vi "ABC Check Move Done.vi"(8 "UART":refnum<vi>, 9 "Response":string, 10 "DataIn":dbl[](array[numeric]), 11 "Data":refnum<vi>) -> (0 "Done":bool, 2 "DataOut":dbl[](array[numeric]), 4 "Position":dbl)   [LabVIEW 2020]
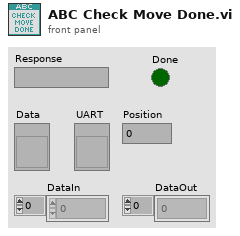
[diagram p1: front panel]
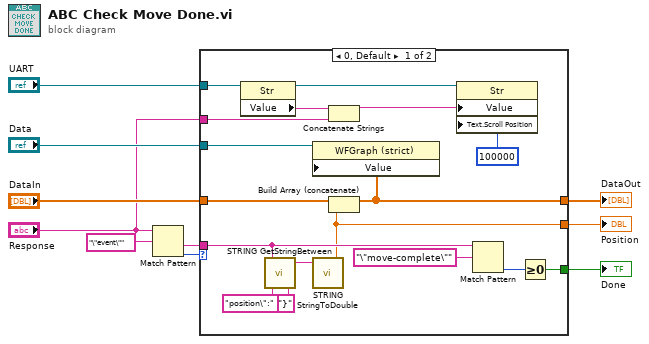
[diagram p0: block diagram]
diagram:
  n1 = Match Pattern(string="Response", regular expression="\"event\"") -> (after substring=w9:string, offset past match=w8:i32)  [unwired: 1 in, 2 out]
  n2 = case shown="0, Default" w8 {
    tunnel: w9 -> [w15 _]
    tunnel: "DataIn" -> [w24 w28]
    tunnel: [w22 w28] -> w6
    tunnel: "Data" -> [w23 _]
    tunnel: "UART" -> [w18 _]
    tunnel: [w14 _] -> w3
    tunnel: "Response" -> [w13 _]
    tunnel: [w11 _] -> w1
    frame 0, Default {
      n3 = property class="Str"(reference=w18) -> (reference out=w12:refnum<vi>, "Value"=w21:string)  [unwired: 1 in, 1 out]
      n4 = call <userlib>:"STRING GetStringBetween.vi"("EndStr"="}", "BeginStr"="position\":", "StrIn"=w15) -> ("StrOut"=w25:string)  [unwired: 2 in]
      n5 = call <userlib>:"STRING StringToDouble.vi"("DblStr"=w25) -> ("Num"=w11:dbl)  [unwired: 4 in]
      n6 = Concatenate Strings(w21, w13) -> (w20:string)
      n7 = Build Array (concatenate)(w24, w11) -> (w22:dbl[])
      n8 = property class="WFGraph (strict)"(reference=w23, "Value"=w22) -> ()  [unwired: 1 in, 2 out]
      n9 = property class="Str"(reference=w12, "Value"=w20, "Text.Scroll Position"=u32 100000) -> ()  [unwired: 1 in, 2 out]
      n10 = Match Pattern(string=w15, regular expression="\"move-complete\"") -> (offset past match=w17:i32)  [unwired: 1 in, 3 out]
      n11 = Greater Or Equal To 0?(x=w17) -> (x >= 0?=w14:bool)
    }
    frame -1 {
    }
  }
  "DataOut" <- w6
  "Done" <- w3
  "Position" <- w1
